vi "Polynomial First Derivitive.vi"(1 "BX":dbl, 2 "CX^2":dbl, 3 "DX^3":dbl, 4 "EX^4":dbl, 5 "FX^5":dbl, 6 "X":dbl) -> (16 "Y":dbl)   [LabVIEW 2015]
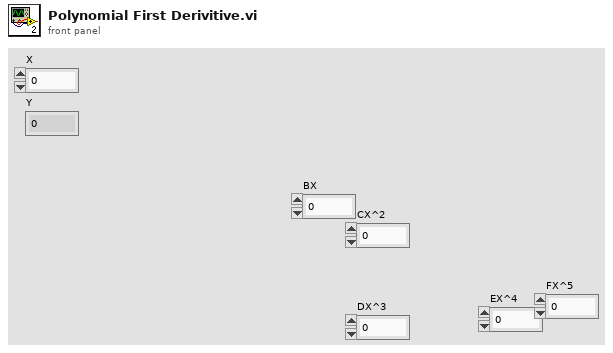
[diagram p1: front panel]
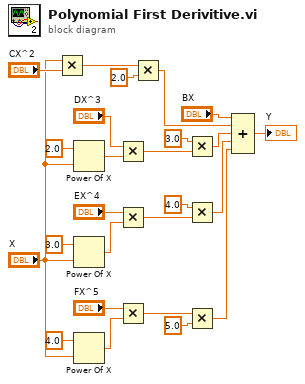
[diagram p0: block diagram]
diagram:
  n1 = Multiply(x="X", y="CX^2") -> (x*y=w15:dbl)
  n2 = Power Of X(1:"X", 2:2.0 ("y")) -> (0:w23:dbl)
  n3 = Power Of X(1:"X", 2:3.0 ("y")) -> (0:w20:dbl)
  n4 = Power Of X(1:"X", 2:4.0 ("y")) -> (0:w17:dbl)
  n5 = Multiply(x="DX^3", y=w23) -> (x*y=w14:dbl)
  n6 = Multiply(x="EX^4", y=w20) -> (x*y=w13:dbl)
  n7 = Multiply(x="FX^5", y=w17) -> (x*y=w12:dbl)
  n8 = Multiply(x=w15, y=2.0) -> (x*y=w8:dbl)
  n9 = Multiply(x=3.0, y=w14) -> (x*y=w6:dbl)
  n10 = Multiply(x=4.0, y=w13) -> (x*y=w4:dbl)
  n11 = Multiply(x=w12, y=5.0) -> (x*y=w2:dbl)
  n12 = Compound Arithmetic op=ADD("BX", w8, w6, w4, w2) -> (→"Y":dbl)
